vi "Periodic Tasks.vi"(8 "error in":errorcluster) -> ()   [LabVIEW 2014]
doc: "This VI runs in parallel to other tasks. It can contain as many user-defined periodic loops as you need. These can carry out PID or other sorts of timed response."
uses:
  <vilib>/Rock Robotics/WPI/Joystick/WPI_JoystickGetSetRefNum.vi
  <vilib>/Rock Robotics/WPI/RobotDrive/WPI_RobotDriveGetSetRefNum.vi
  Global Variables.vi
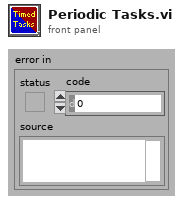
[diagram p1: front panel]
types:
  T1 = typedef "WPI_JoystickDevRef.ctl" = cluster{"Device":T2}
  T2 = typedef "WPI_JoystickDeviceEnum.ctl" = enum16{"USB 0", "USB 1", "USB 2", "USB 3", "USB 4", "USB 5"}
  T3 = typedef "WPI_RobotDriveDevRef.ctl" = cluster{"DevStatus":errorcluster, "Motors[]":T4[], "Square Inputs":bool, "Max Output":dbl}
  T4 = typedef "WPI_MotorControlDeviceRef.ctl" = cluster{"DeviceStatus":errorcluster, "Type":T5, "PWM":cluster{"Controller":T6, "PWM Channel":T7, "DeadBand":T8}, "CAN":cluster{"Device Number":u8, "Control Mode":T9, "Semaphore":T10, "Max Vout":dbl, "TalonSRX Control Mode":T11}, "Invert":bool, "TransformRef":T12, "InvTransformRef":T12}
  T5 = typedef "WPI_MotorControlType.ctl" = enum16{"PWM", "CAN", "CANTalonSRX"}
  T6 = typedef "FPGA_TypedefDigitalModule.ctl" = enum16{"Controller 1"}
  T7 = typedef "FPGA_DIOPWMChannel.ctl" = enum8{"PWM 0", "PWM 1", "PWM 2", "PWM 3", "PWM 4", "PWM 5", "PWM 6", "PWM 7", "PWM 8", "PWM 9", "PWM MXP 0", "PWM MXP 1", "PWM MXP 2", "PWM MXP 3", "PWM MXP 4", "PWM MXP 5", "PWM MXP 6", "PWM MXP 7", "PWM MXP 8", "PWM MXP 9", "Invalid"}
  T8 = typedef "WPI_PWMDeadband.ctl" = cluster{"Name":string, "maxPositivePwm":i32, "minPositivePwm":i32, "centerPwm":i32, "maxNegativePwm":i32, "minNegativePwm":i32, "angularRange":u16}
  T9 = typedef "WPI_CANJaguar_ControlMode.ctl" = enum8{"Percent VBus", "Current", "Speed", "Position", "Voltage"}
  T10 = typedef "Semaphore RefNum" = refnum<k1>
  T11 = typedef "WPI_CANTalonSRX_APIControlMode.ctl" = enum8{"Percent VBus", "Speed", "Position", "Slave", "Unchanged / Invalid"}
  T12 = typedef "WPI_PWMTransform_ConPane.ctl" = refnum<vi>
  T13 = cluster{"JoystickDevRef":T1, "RobotDriveDevRef":T3}
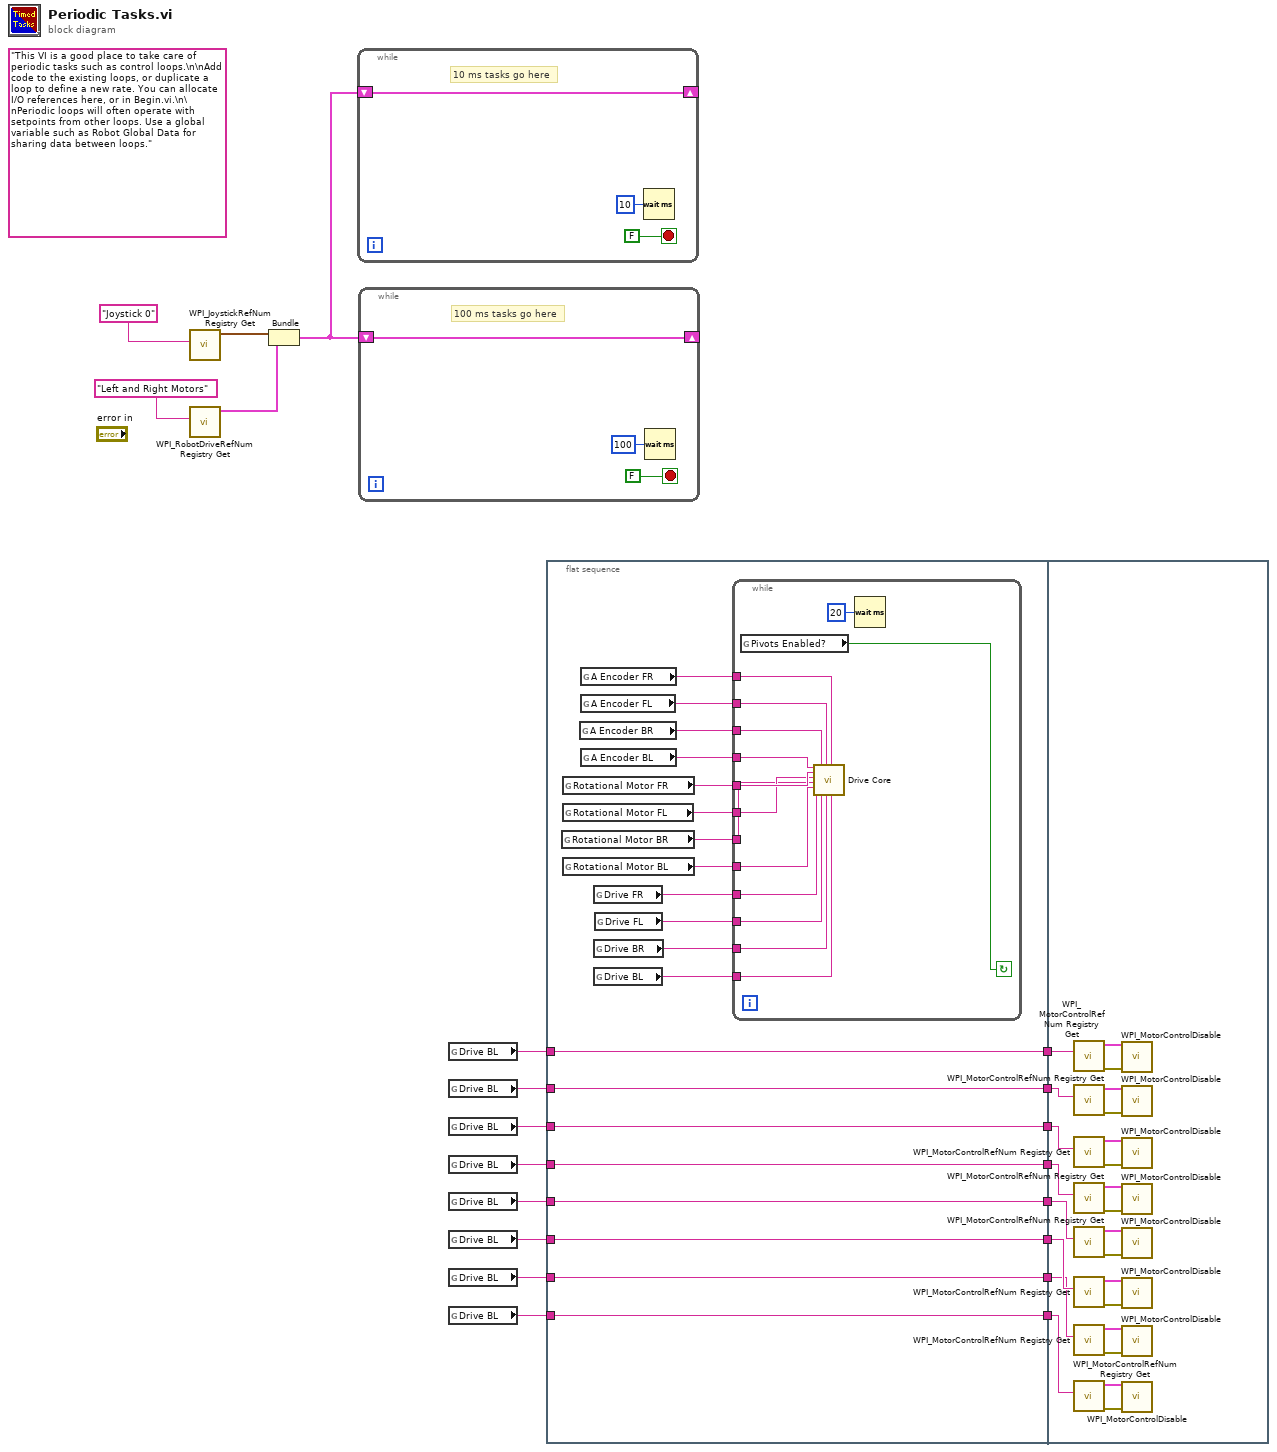
[diagram p0: block diagram]
diagram:
  (unwired) "This VI is a good place to take care of periodic tasks such as control loops.\n\nAdd code to the existing loops, or duplicate a loop to define a new rate. You can allocate I/O references here, or in Begin.vi.\n\nPeriodic loops will often operate with setpoints from other loops. Use a global variable such as Robot Global Data for sharing data between loops."
  n1 = call <vilib>:"WPI_JoystickRefNum Registry Get.vi"("refnum name"="Joystick 0") -> ("JoystickDevRef"=w19:T1)  [unwired: 1 in, 9 out]
  n2 = call <vilib>:"WPI_RobotDriveRefNum Registry Get.vi"("refnum name"="Left and Right Motors") -> ("RobotDriveDevRef"=w18:T3)  [unwired: 1 in, 9 out]
  n3 = Bundle("JoystickDevRef"=w19, "RobotDriveDevRef"=w18) -> (w17:T13)  [unwired: 1 out]
  n4 = while {
    shift-right: [w22] -> _
    shift-left: w17 -> [w22]
    stop <- FALSE stop-if-true
    # "10 ms tasks go here"
    n5 = Wait (ms)(milliseconds to wait=u32 10) -> ()  [unwired: 1 out]
  }
  n6 = while {
    shift-right: [w25] -> _
    shift-left: w17 -> [w25]
    stop <- FALSE stop-if-true
    # "100 ms tasks go here"
    n7 = Wait (ms)(milliseconds to wait=u32 100) -> ()  [unwired: 1 out]
  }
  n8 = global read "Global Variables.vi" "Drive BL"() -> (w15:string)
  n9 = global read "Global Variables.vi" "Drive BL"() -> (w13:string)
  n10 = global read "Global Variables.vi" "Drive BL"() -> (w11:string)
  n11 = global read "Global Variables.vi" "Drive BL"() -> (w9:string)
  n12 = global read "Global Variables.vi" "Drive BL"() -> (w7:string)
  n13 = global read "Global Variables.vi" "Drive BL"() -> (w5:string)
  n14 = global read "Global Variables.vi" "Drive BL"() -> (w3:string)
  n15 = global read "Global Variables.vi" "Drive BL"() -> (w1:string)
  n16 = flat-sequence {
    tunnel: [w35] -> w16
    tunnel: w15 -> [w35]
    tunnel: [w34] -> w14
    tunnel: w13 -> [w34]
    tunnel: [w33] -> w12
    tunnel: w11 -> [w33]
    tunnel: [w32] -> w10
    tunnel: w9 -> [w32]
    tunnel: [w31] -> w8
    tunnel: w7 -> [w31]
    tunnel: [w30] -> w6
    tunnel: w5 -> [w30]
    tunnel: [w29] -> w4
    tunnel: w3 -> [w29]
    tunnel: [w28] -> w2
    tunnel: w1 -> [w28]
    tunnel: w16 -> [w69]
    tunnel: w14 -> [w68]
    tunnel: w12 -> [w67]
    tunnel: w10 -> [w66]
    tunnel: w8 -> [w65]
    tunnel: w6 -> [w64]
    tunnel: w4 -> [w63]
    tunnel: w2 -> [w62]
    frame #0 {
      n17 = global read "Global Variables.vi" "Rotational Motor BR"() -> (w41:string)
      n18 = global read "Global Variables.vi" "Rotational Motor FR"() -> (w43:string)
      n19 = global read "Global Variables.vi" "Rotational Motor FL"() -> (w42:string)
      n20 = global read "Global Variables.vi" "Rotational Motor BL"() -> (w40:string)
      n21 = global read "Global Variables.vi" "A Encoder BR"() -> (w45:string)
      n22 = global read "Global Variables.vi" "A Encoder FR"() -> (w47:string)
      n23 = global read "Global Variables.vi" "A Encoder FL"() -> (w46:string)
      n24 = global read "Global Variables.vi" "A Encoder BL"() -> (w44:string)
      n25 = global read "Global Variables.vi" "Drive FR"() -> (w39:string)
      n26 = global read "Global Variables.vi" "Drive BR"() -> (w37:string)
      n27 = global read "Global Variables.vi" "Drive BL"() -> (w36:string)
      n28 = global read "Global Variables.vi" "Drive FL"() -> (w38:string)
      n29 = while {
        tunnel: w47 -> [w60]
        tunnel: w46 -> [w59]
        tunnel: w45 -> [w58]
        tunnel: w44 -> [w57]
        tunnel: w43 -> [w56]
        tunnel: w42 -> [w55]
        tunnel: w41 -> [w54]
        tunnel: w40 -> [w53]
        tunnel: w39 -> [w52]
        tunnel: w38 -> [w51]
        tunnel: w37 -> [w50]
        tunnel: w36 -> [w49]
        stop <- w61 continue-if-true
        n30 = global read "Global Variables.vi" "Pivots Enabled?"() -> (w61:bool)
        n31 = call "Drive Core.vi"("A Encoder BL"=w57, "Rotational Motor FR"=w56, "Rotational Motor FL"=w55, "Rotational Motor BR"=w54, "Rotational Motor BL"=w53, "Drive Motor FR"=w52, "A Encoder BR"=w58, "Drive Motor FL"=w51, "A Encoder FL"=w59, "Drive Motor BR"=w50, "A Encoder FR"=w60, "Drive Motor BL"=w49) -> ()  [unwired: 8 in]
        n32 = Wait (ms)(milliseconds to wait=u32 20) -> ()  [unwired: 1 out]
      }
    }
    frame #1 {
      n33 = call <vilib>:"WPI_MotorControlRefNum Registry Get.vi"("refnum name"=w69) -> ("error out"=w85:errorcluster, "MotorControlDevRef"=w84:T4)  [unwired: 9 in]
      n34 = call <vilib>:"WPI_MotorControlRefNum Registry Get.vi"("refnum name"=w68) -> ("error out"=w83:errorcluster, "MotorControlDevRef"=w82:T4)  [unwired: 9 in]
      n35 = call <vilib>:"WPI_MotorControlRefNum Registry Get.vi"("refnum name"=w67) -> ("error out"=w81:errorcluster, "MotorControlDevRef"=w80:T4)  [unwired: 9 in]
      n36 = call <vilib>:"WPI_MotorControlRefNum Registry Get.vi"("refnum name"=w66) -> ("error out"=w79:errorcluster, "MotorControlDevRef"=w78:T4)  [unwired: 9 in]
      n37 = call <vilib>:"WPI_MotorControlRefNum Registry Get.vi"("refnum name"=w65) -> ("error out"=w77:errorcluster, "MotorControlDevRef"=w76:T4)  [unwired: 9 in]
      n38 = call <vilib>:"WPI_MotorControlRefNum Registry Get.vi"("refnum name"=w64) -> ("error out"=w75:errorcluster, "MotorControlDevRef"=w74:T4)  [unwired: 9 in]
      n39 = call <vilib>:"WPI_MotorControlRefNum Registry Get.vi"("refnum name"=w63) -> ("error out"=w73:errorcluster, "MotorControlDevRef"=w72:T4)  [unwired: 9 in]
      n40 = call <vilib>:"WPI_MotorControlRefNum Registry Get.vi"("refnum name"=w62) -> ("error out"=w71:errorcluster, "MotorControlDevRef"=w70:T4)  [unwired: 9 in]
      n41 = call <vilib>:"WPI_MotorControlDisable.vi"("error in (no error)"=w85, "MotorControlDevRef"=w84) -> ()  [unwired: 8 in, 2 out]
      n42 = call <vilib>:"WPI_MotorControlDisable.vi"("error in (no error)"=w83, "MotorControlDevRef"=w82) -> ()  [unwired: 8 in, 2 out]
      n43 = call <vilib>:"WPI_MotorControlDisable.vi"("error in (no error)"=w81, "MotorControlDevRef"=w80) -> ()  [unwired: 8 in, 2 out]
      n44 = call <vilib>:"WPI_MotorControlDisable.vi"("error in (no error)"=w79, "MotorControlDevRef"=w78) -> ()  [unwired: 8 in, 2 out]
      n45 = call <vilib>:"WPI_MotorControlDisable.vi"("error in (no error)"=w77, "MotorControlDevRef"=w76) -> ()  [unwired: 8 in, 2 out]
      n46 = call <vilib>:"WPI_MotorControlDisable.vi"("error in (no error)"=w75, "MotorControlDevRef"=w74) -> ()  [unwired: 8 in, 2 out]
      n47 = call <vilib>:"WPI_MotorControlDisable.vi"("error in (no error)"=w73, "MotorControlDevRef"=w72) -> ()  [unwired: 8 in, 2 out]
      n48 = call <vilib>:"WPI_MotorControlDisable.vi"("error in (no error)"=w71, "MotorControlDevRef"=w70) -> ()  [unwired: 8 in, 2 out]
    }
  }
